vi "Motor PWM.vi"(1 "Motor Input 2":refnum<k21>="ConnectorB/DIO2", 2 "Motor Enable":refnum<k21>="ConnectorB/DIO0", 3 "Inside values":T1) -> ()   [LabVIEW 2013]
uses:
  <vilib>/rvi/eio/common/nirviEmuTemplateMethod_errors.vi
  <vilib>/eio/EIONode/EIONode.xnode
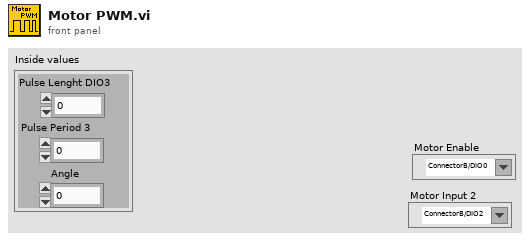
[diagram p1: front panel]
types:
  T1 = cluster{"Pulse Lenght DIO3":i32, "Pulse Period 3":i32, "Angle":i32}
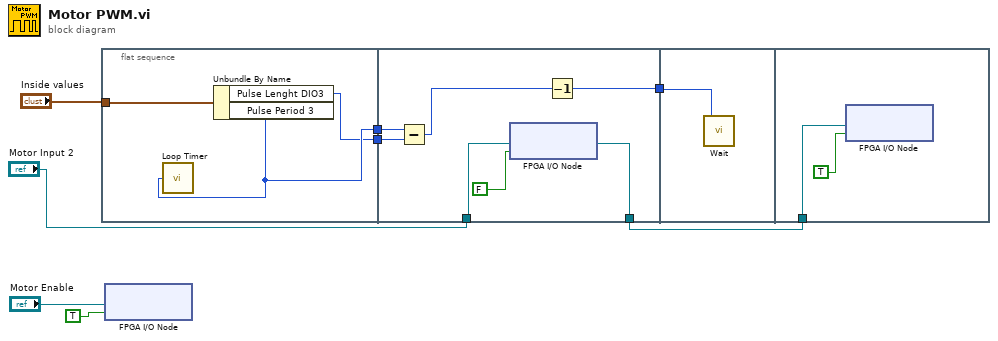
[diagram p0: block diagram]
diagram:
  n1 = flat-sequence {
    tunnel: [w11] -> w8
    tunnel: [w10] -> w7
    tunnel: "Inside values" -> [w9]
    tunnel: [w18] -> w6
    tunnel: w8 -> [w17]
    tunnel: w7 -> [w16]
    tunnel: "Motor Input 2" -> [w14]
    tunnel: [w13] -> w5
    tunnel: w6 -> [w19]
    tunnel: w5 -> [w20]
    frame #0 {
      n2 = Unbundle By Name(w9) -> ("Pulse Lenght DIO3"=w10:i32, "Pulse Period 3"=w11:i32)
      n3 = call "Loop Timer"("Count(Ticks)"=w11) -> ()  [unwired: 1 out]
    }
    frame #1 {
      n4 = Subtract(x=w17, y=w16) -> (x-y=w15:i32)
      n5 = xnode "FPGA I/O Node"("I/O Item"=FALSE ("ConnectorC/DIO7"), "FPGA I/O In"=w14) -> ("FPGA I/O Out"=w13:refnum<k21>)
      n6 = Decrement(x=w15) -> (x-1=w18:i32)
    }
    frame #2 {
      n7 = call "Wait"("Count(Ticks)"=w19) -> ()  [unwired: 1 out]
    }
    frame #3 {
      n8 = xnode "FPGA I/O Node"("I/O Item"=TRUE ("ConnectorC/DIO7"), "FPGA I/O In"=w20) -> ()  [unwired: 1 out]
    }
  }
  n9 = xnode "FPGA I/O Node"("I/O Item"=TRUE ("ConnectorC/DIO7"), "FPGA I/O In"="Motor Enable") -> ()  [unwired: 1 out]
